vi "Read Start Voltage.vi"(0 "Instrument Handle IN":refnum<k15>[](array[refnum]), 5 "Channel Number":string[](array[string]), 7 "Measurement Configuration":T1={"Power Down"=FALSE, "Pin Name"=[], "Source Mode"=[], "Start Value"=[], "Target Value"=[], "Compliance Limit"=[], "Sense Mode"=[], "Default Ramp Rate"=[], "Ramp Rate"=[], "Start Delay"=[], "Relative To"=[], "Transient Response"=[], "Data Capture"=FALSE, "Power line frequency"=1} {"Power line frequency" items=["50 Hz", "60 Hz"]; "Start Value" format="%#_6p"; "Transient Response" items=["Slow", "Normal", "Fast"]; "Sense Mode" items=["Local Sense", "Remote Sense"]; "Relative To" items=["Power sequence start", "Previous source start", "Previous source end"]; "Target Value" format="%#_6p"; "Source Mode" items=["DC Voltage", "DC Current"]; "Start Delay" format="%#_6p"; "Compliance Limit" format="%#_6p"; "Ramp Rate" format="%#_6p"}, 11 "error in (no error)":errorcluster) -> (4 "Instrument Handle OUT":refnum<k15>[](array[refnum]), 6 "Start Value for Power Down":dbl[](array[numeric]), 15 "error out":errorcluster)   [LabVIEW 2024]
uses:
  <instrlib>/niDCPower/nidcpower.llb/niDCPower Output Function.ctl
  <instrlib>/niDCPower/nidcpower.llb/niDCPower Measurement Type.ctl
  controls/Source Mode.ctl
  controls/Relative To.ctl
  controls/Sense Mode.ctl
  Measurement Configuration.ctl
  controls/Transient Response.ctl
  controls/Power line frequency.ctl
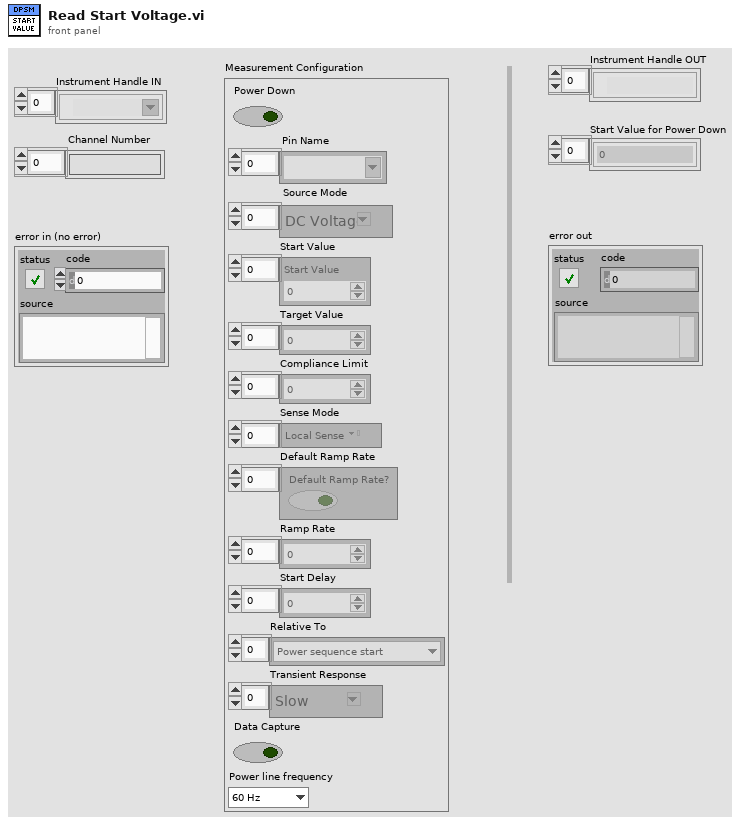
[diagram p1: front panel]
types:
  T1 = typedef "devicePowerSequencingModule.lvlib/Measurement Configuration.ctl" = cluster{"Power Down":bool, "Pin Name":string[], "Source Mode":T2[], "Start Value":dbl[], "Target Value":dbl[], "Compliance Limit":dbl[], "Sense Mode":T3[], "Default Ramp Rate":bool[], "Ramp Rate":dbl[], "Start Delay":dbl[], "Relative To":T4[], "Transient Response":T5[], "Data Capture":bool, "Power line frequency":T6}
  T2 = typedef "devicePowerSequencingModule.lvlib/Source Mode.ctl" = i32
  T3 = typedef "devicePowerSequencingModule.lvlib/Sense Mode.ctl" = i32
  T4 = typedef "devicePowerSequencingModule.lvlib/Relative To.ctl" = u32
  T5 = typedef "devicePowerSequencingModule.lvlib/Transient Response.ctl" = i32
  T6 = typedef "devicePowerSequencingModule.lvlib/Power line frequency.ctl" = u32
  T7 = typedef "niDCPower Measurement Type.ctl" = i32
  T8 = typedef "niDCPower Output Function.ctl" = i32
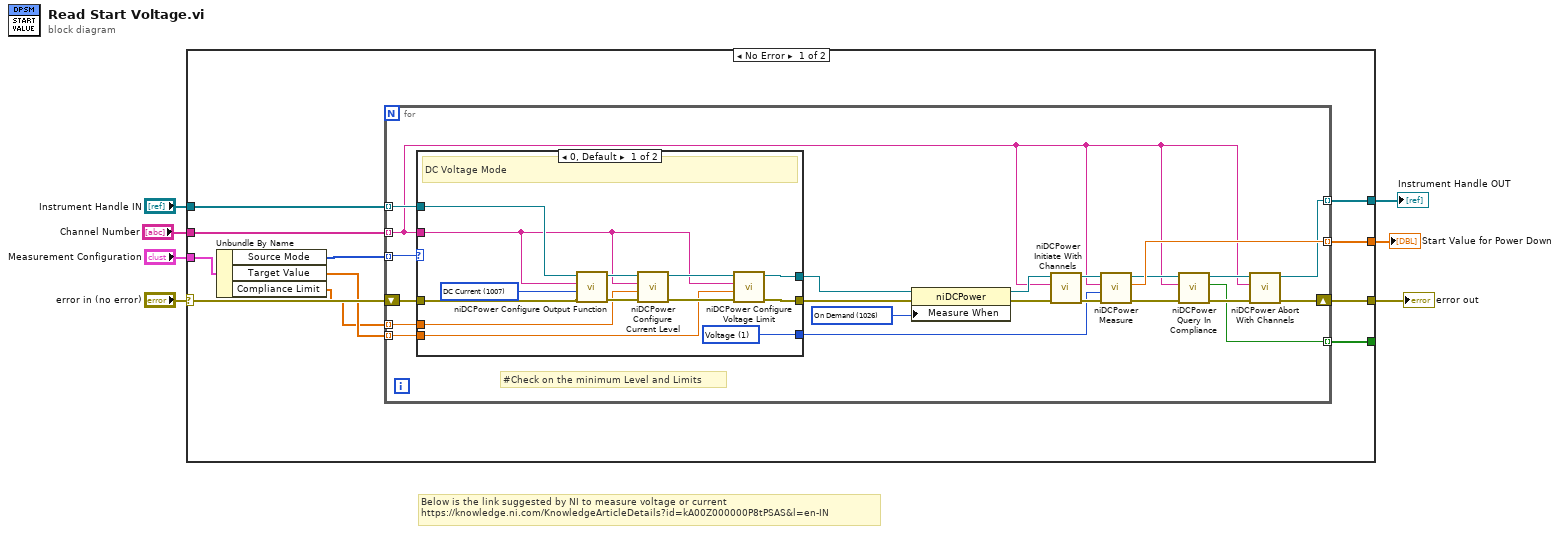
[diagram p0: block diagram]
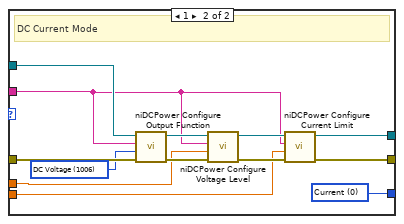
[diagram p2: hidden frame]
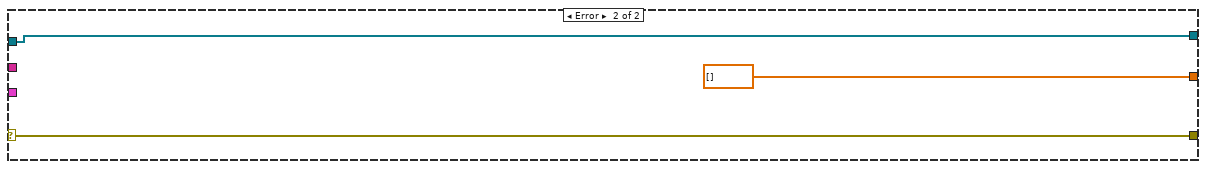
[diagram p3: hidden frame]
diagram:
  # "Below is the link suggested by NI to measure voltage or current\nhttps://knowledge.ni.com/KnowledgeArticleDetails?id=kA00Z000000P8tPSAS&l=en-IN"
  n1 = case shown="No Error" "error in (no error)" {
    selector: "error in (no error)" -> [w15 w68]
    tunnel: "Instrument Handle IN" -> [w18 w67]
    tunnel: "Measurement Configuration" -> [w17 _]
    tunnel: [w14 w68] -> w4
    tunnel: [w13 dbl[] []] -> w3
    tunnel: "Channel Number" -> [w12 _]
    tunnel: [w10 w67] -> w1
    tunnel: [w8 _] -> _
    frame No Error {
      n2 = Unbundle By Name(w17) -> ("Source Mode"=w16:T2[], "Target Value"=w11:dbl[], "Compliance Limit"=w9:dbl[])
      n3 = for {
        tunnel: w18 -> [w38] mode=indexing
        tunnel: w16 -> [w40] mode=indexing
        tunnel: [w29] -> w13 mode=indexing
        shift-right: [w27] -> w14
        shift-left: w15 -> [w39]
        tunnel: w12 -> [w21] mode=indexing
        tunnel: w11 -> [w28] mode=indexing
        tunnel: [w26] -> w10 mode=indexing
        tunnel: w9 -> [w25] mode=indexing
        tunnel: [w19] -> w8 mode=indexing
        w35 = 1026 items=["Automatically after Source Complete"=1025, "On Demand"=1026, "On Measure Trigger"=1027] ("Measurement:Advanced:Measure When")
        # "#Check on the minimum Level and Limits"
        n4 = case shown="0, Default" w40 {
          tunnel: w39 -> [w53 w66]
          tunnel: w38 -> [w47 w61]
          tunnel: [w46 w59] -> w36
          tunnel: [w45 w58] -> w37
          tunnel: [w44 w57] -> w30
          tunnel: w21 -> [w43 w56]
          tunnel: w28 -> [w41 w55]
          tunnel: w25 -> [w42 w54]
          frame 0, Default {
            w44 = T7 1 items=["Current", "Voltage"] ("measurement type")
            w52 = T8 1007 items=["DC Voltage"=1006, "DC Current"=1007, "Pulse Voltage"=1049, "Pulse Current"=1050] ("output function")
            # "DC Voltage Mode"
            n5 = call <instrlib>:"niDCPower Configure Output Function.vi"("error in (no error)"=w53, "output function"=w52, "channel name"=w43, "instrument handle"=w47) -> ("error out"=w48:errorcluster, "instrument handle out"=w49:refnum<k15>)  [unwired: 6 in]
            n6 = call <instrlib>:"niDCPower Configure Current Level.vi"("error in (no error)"=w48, "current level"=w42, "channel name"=w43, "instrument handle"=w49) -> ("error out"=w51:errorcluster, "instrument handle out"=w50:refnum<k15>)  [unwired: 6 in]
            n7 = call <instrlib>:"niDCPower Configure Voltage Limit.vi"("error in (no error)"=w51, "voltage limit"=w41, "channel name"=w43, "instrument handle"=w50) -> ("error out"=w45:errorcluster, "instrument handle out"=w46:refnum<k15>)  [unwired: 6 in]
          }
          frame 1 {
            w57 = T7 0 items=["Current", "Voltage"] ("measurement type")
            w65 = T8 1006 items=["DC Voltage"=1006, "DC Current"=1007, "Pulse Voltage"=1049, "Pulse Current"=1050] ("output function")
            # "DC Current Mode"
            n8 = call <instrlib>:"niDCPower Configure Output Function.vi"("error in (no error)"=w66, "output function"=w65, "channel name"=w56, "instrument handle"=w61) -> ("error out"=w64:errorcluster, "instrument handle out"=w62:refnum<k15>)  [unwired: 6 in]
            n9 = call <instrlib>:"niDCPower Configure Voltage Level.vi"("error in (no error)"=w64, "voltage level"=w54, "channel name"=w56, "instrument handle"=w62) -> ("error out"=w63:errorcluster, "instrument handle out"=w60:refnum<k15>)  [unwired: 6 in]
            n10 = call <instrlib>:"niDCPower Configure Current Limit.vi"("error in (no error)"=w63, "current limit"=w55, "channel name"=w56, "instrument handle"=w60) -> ("error out"=w58:errorcluster, "instrument handle out"=w59:refnum<k15>)  [unwired: 6 in]
          }
        }
        n11 = property class="niDCPower"(reference=w36, error in=w37, "Measure When"=w35) -> (reference out=w33:refnum<k15>, error out=w34:errorcluster)
        n12 = call <instrlib>:"niDCPower Initiate With Channels.vi"("error in (no error)"=w34, "channel name"=w21, "instrument handle"=w33) -> ("error out"=w31:errorcluster, "instrument handle out"=w32:refnum<k15>)  [unwired: 7 in]
        n13 = call <instrlib>:"niDCPower Measure.vi"("error in (no error)"=w31, "measurement type"=w30, "channel name"=w21, "instrument handle"=w32) -> ("error out"=w22:errorcluster, "measurement"=w29:dbl, "instrument handle out"=w24:refnum<k15>)  [unwired: 5 in]
        n14 = call <instrlib>:"niDCPower Query In Compliance.vi"("error in (no error)"=w22, "channel name"=w21, "instrument handle"=w24) -> ("error out"=w20:errorcluster, "in compliance?"=w19:bool, "instrument handle out"=w23:refnum<k15>)  [unwired: 6 in]
        n15 = call <instrlib>:"niDCPower Abort With Channels.vi"("error in (no error)"=w20, "channel name"=w21, "instrument handle"=w23) -> ("error out"=w27:errorcluster, "instrument handle out"=w26:refnum<k15>)  [unwired: 7 in]
      }
    }
    frame Error {
    }
  }
  "error out" <- w4
  "Start Value for Power Down" <- w3
  "Instrument Handle OUT" <- w1
